vi "TrackExtractor.vi"() -> ()   [LabVIEW 2012]
panel:
  out "error out":errorcluster
  in  "Tracking file":path=path "C:/Users/Ludovico/Lavoro/Experiments/Autofocus/vermi/track3.txt"
  in  "Interframe time (s)":dbl=0.1
  in  "Positions file":path=path "C:/Users/Ludovico/Lavoro/Experiments/Autofocus/vermi/CONFSTAGELOG/2016_12_16_10_06.txt"
  in  "error in (no error)":errorcluster
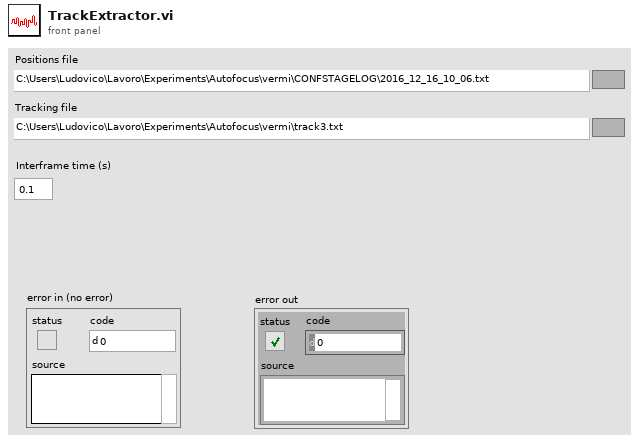
[diagram p1: front panel]
types:
  T1 = cluster{"Object Center":cluster{"X":sgl, "Y":sgl}, "Bounding Box":cluster{"X Left":i32, "Y Top":i32, "X Right":i32, "Y Bottom":i32}, "Area":sgl, "Orientation":sgl, "Aspect Ratio":sgl, "Nb Holes":i32}[]
  T2 = cluster{"X":dbl[], "Y":dbl[], "Focus":dbl[], "Time array":dbl[]}
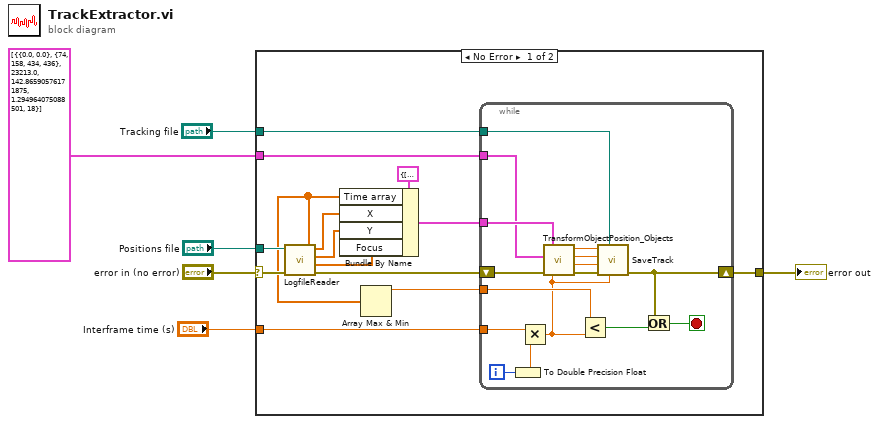
[diagram p0: block diagram]
diagram:
  n1 = case shown="No Error" "error in (no error)" {
    selector: "error in (no error)" -> [w16 _]
    tunnel: "Positions file" -> [w15 _]
    tunnel: "Interframe time (s)" -> [w14 _]
    tunnel: T1 [{"Object Center"={"X"=0.0, "Y"=0.0}, "Bounding Box"={"X Left"=74, "Y Top"=158, "X Right"=434, "Y Bottom"=436}, "Area"=23213.0, "Orientation"=142.8659, "Aspect Ratio"=1.2949641, "Nb Holes"=18}] ("Objects") -> [w9 _]
    tunnel: "Tracking file" -> [w8 _]
    tunnel: [w7 _] -> w1
    frame No Error {
      n2 = call "LogfileReader.vi"("error in (no error)"=w16, "Positions file"=w15) -> ("error out"=w13:errorcluster, "Focus"=w17:dbl[], "Y"=w18:dbl[], "X"=w19:dbl[], "Time"=w12:dbl[])  [unwired: 5 in]
      n3 = Bundle By Name(cluster=T2 {"X"=[], "Y"=[], "Focus"=[], "Time array"=[]} ("Spacetime cluster"), "Time array"=w12, "X"=w19, "Y"=w18, "Focus"=w17) -> (w10:T2)
      n4 = Array Max & Min(array=w12) -> (max value=w11:dbl)  [unwired: 3 out]
      n5 = while {
        tunnel: w14 -> [w35]
        shift-right: [w30] -> w7
        shift-left: w13 -> [w29]
        tunnel: w11 -> [w33]
        tunnel: w10 -> [w27]
        tunnel: w9 -> [w26]
        tunnel: w8 -> [w22]
        i -> [w36]
        stop <- w31 stop-if-true
        n6 = To Double Precision Float(number=w36) -> (double precision float=w34:dbl)
        n7 = Multiply(x=w35, y=w34) -> (x*y=w21:dbl)
        n8 = call "TransformObjectPosition_Objects.vi"("Image time"=w21, "error in (no error)"=w29, "Objects (pixel)"=w26, "Spacetime cluster"=w27) -> ("error out"=w28:errorcluster, "Focus out"=w23:dbl, "Y out"=w24:dbl, "X out"=w25:dbl)  [unwired: 4 in]
        n9 = Less?(x=w33, y=w21) -> (x < y?=w32:bool)
        n10 = call "SaveTrack.vi"("Time"=w21, "Track file"=w22, "error in (no error)"=w28, "Focus"=w23, "Y"=w24, "X"=w25) -> ("error out"=w30:errorcluster)  [unwired: 5 in]
        n11 = Or(x=w30, y=w32) -> (x .or. y?=w31:bool)
      }
    }
    frame Error {
    }
  }
  "error out" <- w1
